vi "User Selected Load Size.vi"(6 "User Selected Load Size":T1=enum."Super", 8 "Error In":errorcluster, 9 "GEA Inputs":T2 {"Destination" format="%.0x"; "Source" format="%.0x"}, 10 "Standalone?":bool, 11 "GEA2 Reference In":refnum<k24>) -> (0 "Error Out":errorcluster, 3 "GEA2 Reference Out":refnum<k24>)   [LabVIEW 2016, in "TLMB.lvlib"]
uses:
  Projects/TLMB.lvlib
  Q:/Common/DLLs/GEA3/GeaCommunication.dll
  Common/DLLs/GEA3/GeaCommunication.dll
  Common/LabVIEW GEA2 Toolkit/LabVIEW_GEA2_Toolkit.lvlibp/type defs/Source_Destination.ctl
  type defs/User Selected Load Size.ctl
  Common/LabVIEW GEA2 Toolkit/LabVIEW_GEA2_Toolkit.lvlibp/type defs/ERD Write Data In.ctl
  Common/LabVIEW GEA2 Toolkit/LabVIEW_GEA2_Toolkit.lvlibp/type defs/Data Type.ctl
  Common/LabVIEW GEA2 Toolkit/LabVIEW_GEA2_Toolkit.lvlibp
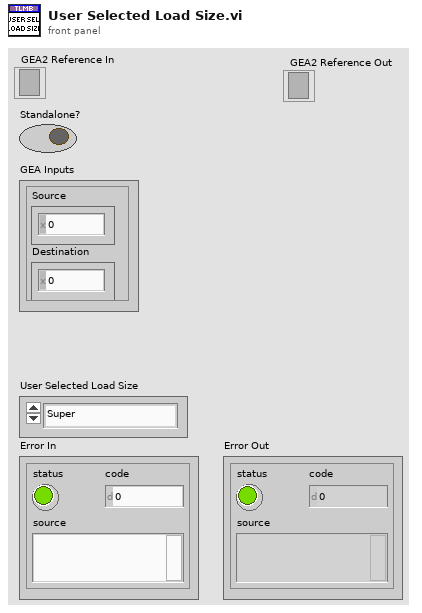
[diagram p1: front panel]
types:
  T1 = typedef "TLMB.lvlib/User Selected Load Size.ctl" = enum16{"Small", "Medium", "Large", "Super"}
  T2 = typedef "LabVIEW_GEA2_Toolkit.lvlibp/Source_Destination.ctl" = cluster{"Source":u8, "Destination":u8}
  T3 = typedef "LabVIEW_GEA2_Toolkit.lvlibp/ERD Write Data In.ctl" = cluster{"ERD Number":u16, "Data Type":T4, "Data":string}
  T4 = typedef "LabVIEW_GEA2_Toolkit.lvlibp/Data Type.ctl" = enum16{"string", "boolean", "uint8_t", "uint16_t", "uint32_t", "uint64_t", "int8_t", "int16_t", "int32_t", "int64_t"}
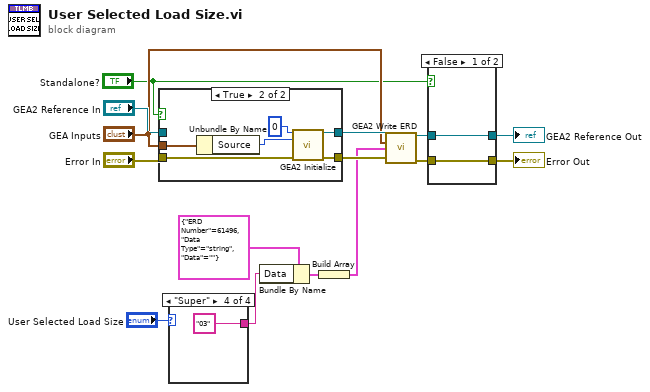
[diagram p0: block diagram]
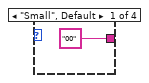
[diagram p2: hidden frame]
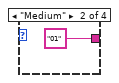
[diagram p3: hidden frame]
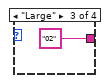
[diagram p4: hidden frame]
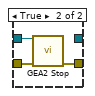
[diagram p5: hidden frame]
diagram:
  n1 = case shown="True" "Standalone?" {
    tunnel: "Error In" -> [w16 w23]
    tunnel: [w16 w22] -> w15
    tunnel: "GEA2 Reference In" -> [w17 _]
    tunnel: [w17 w21] -> w10
    tunnel: "GEA Inputs" -> [_ w19]
    frame False {
    }
    frame True {
      n2 = Unbundle By Name(w19) -> ("Source"=w20:u8)
      n3 = call "GEA2 Initialize.vi"("Board Index"=0, "Source Address"=w20, "error in"=w23) -> ("GEA2 Reference Out"=w21:refnum<k24>, "error out"=w22:errorcluster)  [unwired: 10 in, 1 out]
    }
  }
  n4 = case shown="\"Super\"" "User Selected Load Size" {
    tunnel: ["00" "01" "02" "03"] -> w6
    frame "Small", Default {
    }
    frame "Medium" {
    }
    frame "Large" {
    }
    frame "Super" {
    }
  }
  n5 = Bundle By Name(cluster=T3 {"ERD Number"=61496, "Data Type"=enum."string", "Data"=""} ("ERD Write Data In"), "Data"=w6) -> (w7:T3)
  n6 = Build Array(w7) -> (w1:T3[])
  n7 = call "GEA2 Write ERD.vi"("GEA2 Reference In"=w10, "GEA Inputs"="GEA Inputs", "Write ERD List"=w1, "Error In"=w15) -> ("GEA2 Reference Out"=w4:refnum<k24>, "Error Out"=w3:errorcluster)  [unwired: 9 in, 1 out]
  n8 = case shown="False" "Standalone?" {
    tunnel: w3 -> [w28 w32]
    tunnel: [w28 w31] -> w13
    tunnel: w4 -> [w29 w30]
    tunnel: [w29 _] -> w11
    frame False {
    }
    frame True {
      n9 = call "GEA2 Stop.vi"("GEA2 Reference In"=w30, "Error In"=w32) -> ("Error Out"=w31:errorcluster)  [unwired: 13 in]
    }
  }
  "Error Out" <- w13
  "GEA2 Reference Out" <- w11
